vi "PLC.Dial800.Build OPC URL.vi"(8 "error in (no error)":errorcluster, 10 "OPC Server":T3={"IP"="localhost", "Topic"="Stn800", "Server"="RSLinx OPC Server", "VarRoot"="Program:Stn001_90_OffloadMain", "TestPCArray"="TestPC", "VarNames"={"SN"="SN", "Reset"="Reset", "HeartbeatPLC"="HeartbeatPLC", "HeartbeatPC"="HeartbeatTestPC", "Start"="Start", "Running"="Running", "Done"="Done", "Pass"="Pass"}}, 11 "Nest":i32) -> (0 "error out":errorcluster, 3 "Var URLs":T1[](array[typedef]))   [LabVIEW 2018]
uses:
  PLC.Dial800.OPC Server Config.ctl
  PLC.Dial800.VarNames.ctl
  PLC.Dial800.Var URL Item.ctl
  PLC.Dial800.VarNameSelector.ctl
panel:
  # "(Access path)"
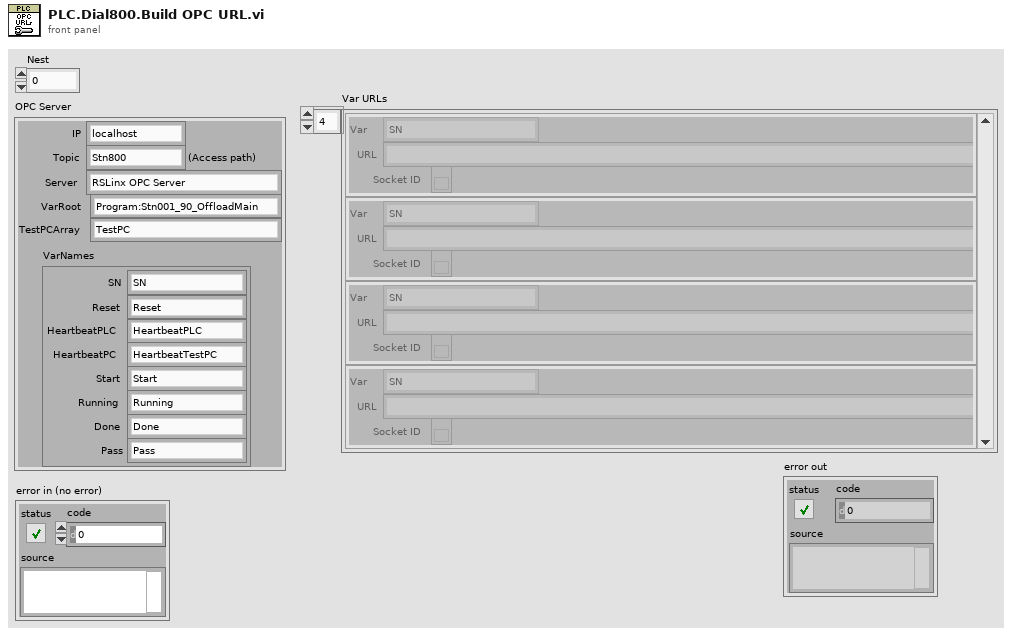
[diagram p1: front panel]
types:
  T1 = typedef "PLC.Dial800.Var URL Item.ctl" = cluster{"Var":T2, "URL":string, "Socket ID":refnum<k13>}
  T2 = typedef "PLC.Dial800.VarNameSelector.ctl" = enum16{"SN", "Reset", "HeartBeat_PLC", "Heartbeat_PC", "Start", "Running", "Done", "Pass"}
  T3 = typedef "PLC.Dial800.OPC Server Config.ctl" = cluster{"IP":string, "Topic":string, "Server":string, "VarRoot":string, "TestPCArray":string, "VarNames":T4}
  T4 = typedef "PLC.Dial800.VarNames.ctl" = cluster{"SN":string, "Reset":string, "HeartbeatPLC":string, "HeartbeatPC":string, "Start":string, "Running":string, "Done":string, "Pass":string}
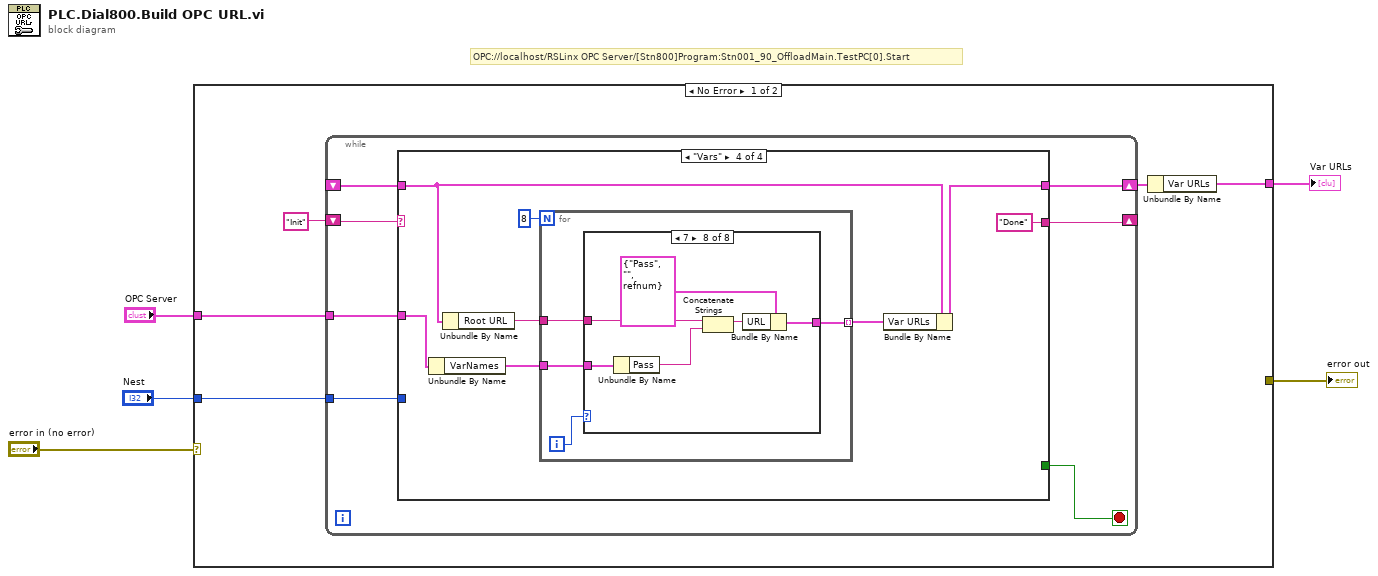
[diagram p0: block diagram]
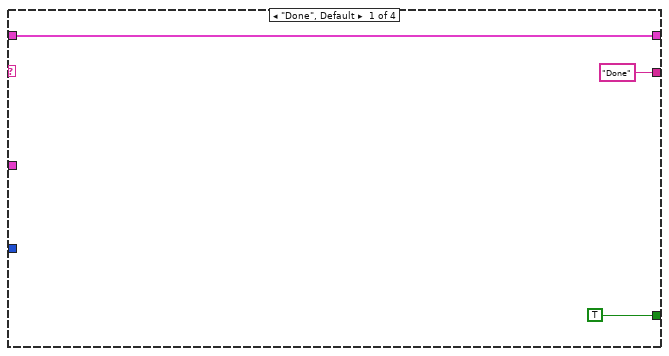
[diagram p2: hidden frame]
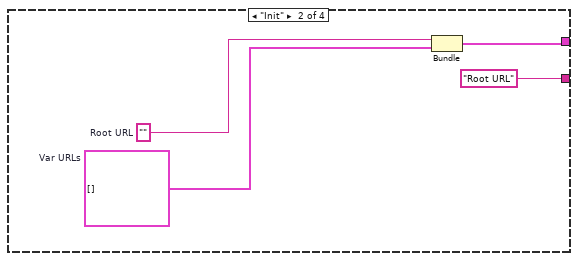
[diagram p3: hidden frame]
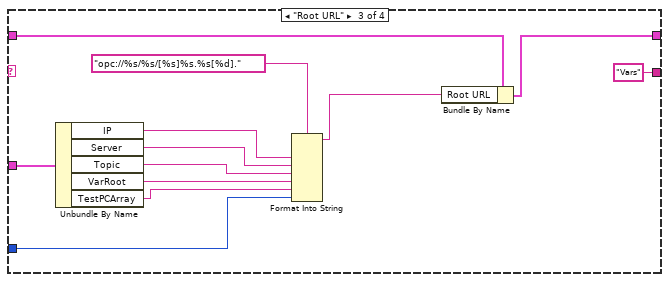
[diagram p4: hidden frame]
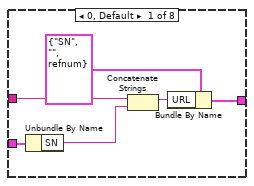
[diagram p5: hidden frame]
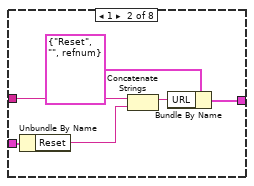
[diagram p6: hidden frame]
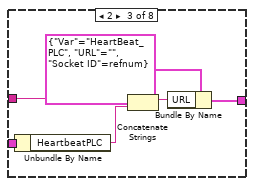
[diagram p7: hidden frame]
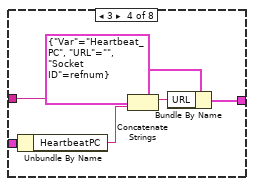
[diagram p8: hidden frame]
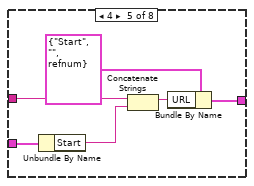
[diagram p9: hidden frame]
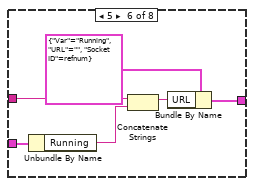
[diagram p10: hidden frame]
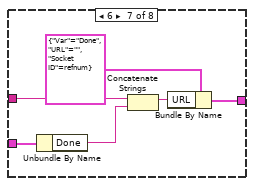
[diagram p11: hidden frame]
diagram:
  # "OPC://localhost/RSLinx OPC Server/[Stn800]Program:Stn001_90_OffloadMain.TestPC[0].Start"
  n1 = case shown="No Error" "error in (no error)" {
    selector: "error in (no error)" -> [_ w97]
    tunnel: [_ w97] -> w4
    tunnel: "Nest" -> [w9 _]
    tunnel: "OPC Server" -> [w8 _]
    tunnel: [w6 _] -> w1
    frame No Error {
      n2 = while {
        shift-right: [w13] -> w7
        shift-left: _ -> [w14]
        shift-right: [w15] -> _
        shift-left: "Init" -> [w17]
        tunnel: w9 -> [w12]
        tunnel: w8 -> [w11]
        stop <- w16 stop-if-true
        n3 = case shown="\"Vars\"" w17 {
          tunnel: [TRUE _ _ _] -> w16
          tunnel: ["Done" "Root URL" "Vars" "Done"] -> w15
          tunnel: w14 -> [w18 _ w33 w41]
          tunnel: [w18 w22 w32 w42] -> w13
          tunnel: w12 -> [_ _ w25 _]
          tunnel: w11 -> [_ _ w35 w43]
          frame "Done", Default {
          }
          frame "Init" {
            w24 = ""  # Root URL
            w23 = T1[] []  # Var URLs
            n4 = Bundle("Root URL"=w24, "Var URLs"=w23) -> (w22:cluster{"Root URL":string, "Var URLs":T1[]})  [unwired: 1 in]
          }
          frame "Root URL" {
            n5 = Unbundle By Name(w35) -> ("IP"=w30:string, "Server"=w29:string, "Topic"=w28:string, "VarRoot"=w27:string, "TestPCArray"=w26:string)
            n6 = Format Into String(format string="opc://%s/%s/[%s]%s.%s[%d].", w30, w29, w28, w27, w26, w25) -> (resulting string=w31:string)  [unwired: 2 in, 1 out]
            n7 = Bundle By Name(cluster=w33, "Root URL"=w31) -> (w32:cluster{"Root URL":string, "Var URLs":T1[]})
          }
          frame "Vars" {
            n8 = Unbundle By Name(w43) -> ("VarNames"=w39:T4)
            n9 = Unbundle By Name(w41) -> ("Root URL"=w40:string)
            n10 = for {
              N: 8 -> [_]
              tunnel: w40 -> [w48]
              tunnel: w39 -> [w47]
              tunnel: [w45] -> w38 mode=indexing
              i -> [w46]
              n11 = case shown="7" w46 {
                tunnel: w48 -> [w54 w60 w66 w72 w78 w84 w90 w96]
                tunnel: w47 -> [w53 w59 w65 w71 w77 w83 w89 w95]
                tunnel: [w49 w55 w61 w67 w73 w79 w85 w91] -> w45
                frame 0, Default {
                  n12 = Unbundle By Name(w53) -> ("SN"=w52:string)
                  n13 = Concatenate Strings(w54, w52) -> (w50:string)
                  n14 = Bundle By Name(cluster=T1 {"Var"=enum."SN", "URL"="", "Socket ID"=refnum} ("Var URL Item"), "URL"=w50) -> (w49:T1)
                }
                frame 1 {
                  n15 = Unbundle By Name(w59) -> ("Reset"=w58:string)
                  n16 = Concatenate Strings(w60, w58) -> (w56:string)
                  n17 = Bundle By Name(cluster=T1 {"Var"=enum."Reset", "URL"="", "Socket ID"=refnum} ("Var URL Item"), "URL"=w56) -> (w55:T1)
                }
                frame 2 {
                  n18 = Unbundle By Name(w65) -> ("HeartbeatPLC"=w64:string)
                  n19 = Concatenate Strings(w66, w64) -> (w62:string)
                  n20 = Bundle By Name(cluster=T1 {"Var"=enum."HeartBeat_PLC", "URL"="", "Socket ID"=refnum} ("Var URL Item"), "URL"=w62) -> (w61:T1)
                }
                frame 3 {
                  n21 = Unbundle By Name(w71) -> ("HeartbeatPC"=w70:string)
                  n22 = Concatenate Strings(w72, w70) -> (w68:string)
                  n23 = Bundle By Name(cluster=T1 {"Var"=enum."Heartbeat_PC", "URL"="", "Socket ID"=refnum} ("Var URL Item"), "URL"=w68) -> (w67:T1)
                }
                frame 4 {
                  n24 = Unbundle By Name(w77) -> ("Start"=w76:string)
                  n25 = Concatenate Strings(w78, w76) -> (w74:string)
                  n26 = Bundle By Name(cluster=T1 {"Var"=enum."Start", "URL"="", "Socket ID"=refnum} ("Var URL Item"), "URL"=w74) -> (w73:T1)
                }
                frame 5 {
                  n27 = Unbundle By Name(w83) -> ("Running"=w82:string)
                  n28 = Concatenate Strings(w84, w82) -> (w80:string)
                  n29 = Bundle By Name(cluster=T1 {"Var"=enum."Running", "URL"="", "Socket ID"=refnum} ("Var URL Item"), "URL"=w80) -> (w79:T1)
                }
                frame 6 {
                  n30 = Unbundle By Name(w89) -> ("Done"=w88:string)
                  n31 = Concatenate Strings(w90, w88) -> (w86:string)
                  n32 = Bundle By Name(cluster=T1 {"Var"=enum."Done", "URL"="", "Socket ID"=refnum} ("Var URL Item"), "URL"=w86) -> (w85:T1)
                }
                frame 7 {
                  n33 = Unbundle By Name(w95) -> ("Pass"=w94:string)
                  n34 = Concatenate Strings(w96, w94) -> (w92:string)
                  n35 = Bundle By Name(cluster=T1 {"Var"=enum."Pass", "URL"="", "Socket ID"=refnum} ("Var URL Item"), "URL"=w92) -> (w91:T1)
                }
              }
            }
            n36 = Bundle By Name(cluster=w41, "Var URLs"=w38) -> (w42:cluster{"Root URL":string, "Var URLs":T1[]})
          }
        }
      }
      n37 = Unbundle By Name(w7) -> ("Var URLs"=w6:T1[])
    }
    frame Error {
    }
  }
  "error out" <- w4
  "Var URLs" <- w1
